vi "Counter - Count Edges AVG.vi"(6 "zero lag +":i32=1, 8 "AC length":i32, 10 "Sample Rate":dbl=100000.0, 11 "Total Time (s)":i32=100) -> (1 "G2 MultipTau":dbl[][](graph), 2 "output params":T1, 3 "N":i32, 5 "Cancel Button out":bool)   [LabVIEW 2022 SP3]
doc: "This example demonstrates how to continuously read back the number of digital edges that have been counted by a counter input. It uses an external clock so that the samples of the count register occur at regular intervals. If you do not need deterministic sampling of the count register, refer instead to the Count Edges example which does not use an external clock.\n\nFor instructions on how to connect your signals to the DAQ device, refer to your device documentation."
uses:
  <vilib>/DAQmx/read.llb/DAQmx Read (Counter 1D U32 1Chan NSamp).vi
  <vilib>/DAQmx/create/channels.llb/DAQmx Create Channel (CO-Pulse Generation-Frequency).vi
  <vilib>/DAQmx/configure/timing.llb/DAQmx Timing (Implicit).vi
  <vilib>/DAQmx/create/channels.llb/DAQmx Create Channel (CI-Count Edges).vi
  <vilib>/DAQmx/configure/timing.llb/DAQmx Timing (Sample Clock).vi
  <vilib>/DAQmx/miscellaneous.llb/DAQmx Fill In Error Info.vi
  <resource>/objmgr/daqmx.rc
panel:
  out "Current N":i32
  in  "Cancel Button":bool
  in  "Input Terminal":tag="/Dev1/PFI3"
  in  "Counter":tag="Dev1/ctr1"
  in  "Sample Clock Source":tag="/Dev1/PFI12"
  # "Channel Settings"
  # "Timing Settings"
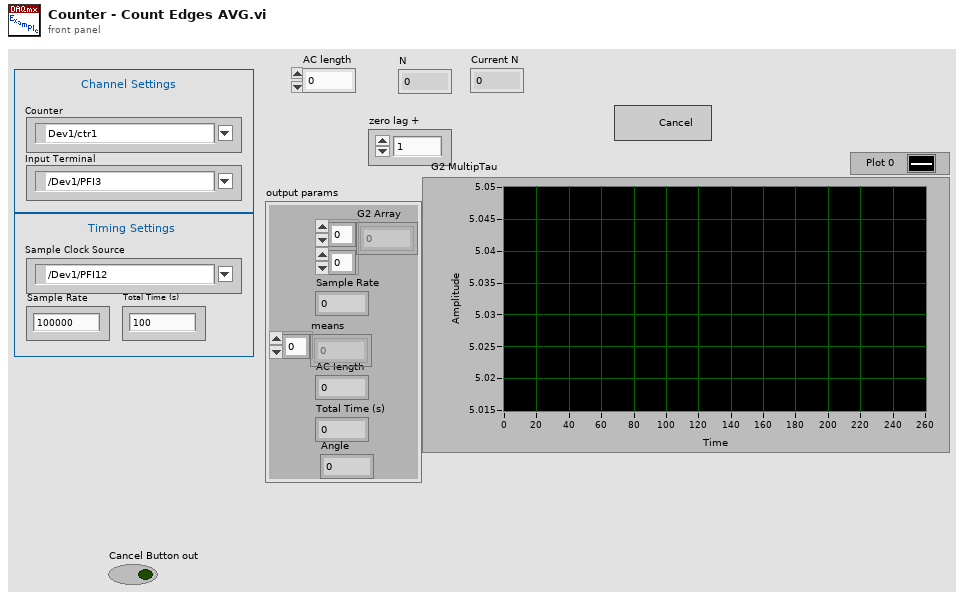
[diagram p1: front panel]
types:
  T1 = cluster{"G2 Array":dbl[][], "Sample Rate":dbl, "means":dbl[], "AC length":i32, "Total Time (s)":i32, "Angle":dbl}
  T2 = cluster{"Data out":dbl[][], "Sample Rate":dbl, dbl[], "AC length":i32, "Total Time (s)":i32, "AC length":dbl}
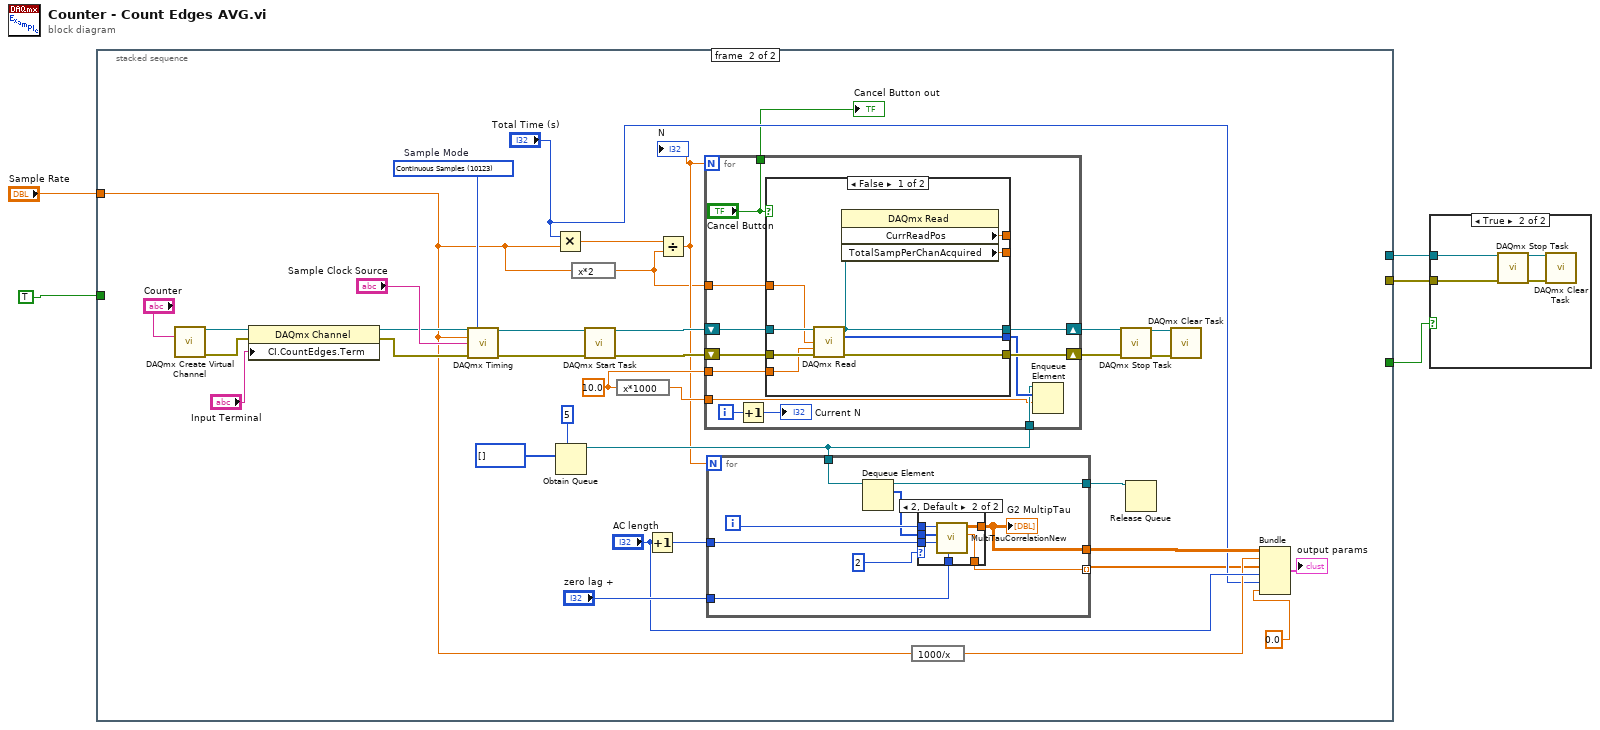
[diagram p0: block diagram]
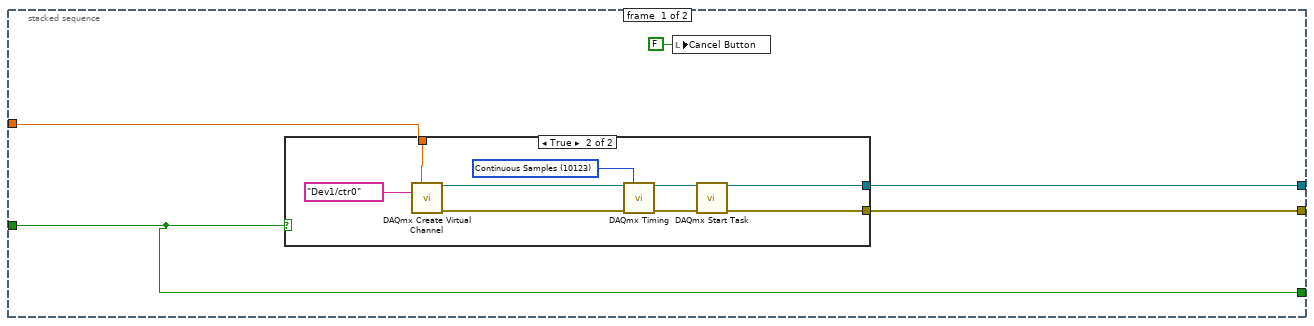
[diagram p2: hidden frame]
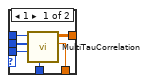
[diagram p4: hidden frame]
diagram:
  n1 = stacked-sequence {
    tunnel: TRUE -> [w6 _]
    tunnel: "Sample Rate" -> [w8 w22]
    tunnel: [w10 _] -> w4
    tunnel: [w9 _] -> w3
    tunnel: [w6 _] -> w1
    frame #0 {
      n2 = case shown="True" w6 {
        tunnel: w8 -> [_ w19]
        tunnel: [_ w17] -> w10
        tunnel: [_ w16] -> w9
        frame False {
        }
        frame True {
          w13 = 10123 items=["Finite Samples"=10178, "Continuous Samples"=10123, "Hardware Timed Single Point"=12522] ("sample mode")
          n3 = call-poly <vilib>:"DAQmx Create Virtual Channel.vi"("frequency"=w19, "counter"=tag "Dev1/ctr0") -> ("task out"=w15:refnum<k21>, "error out"=w12:errorcluster)  [unwired: 12 in]
          n4 = call-poly <vilib>:"DAQmx Timing.vi"("task/channels in"=w15, "sample mode"=w13, "error in"=w12) -> ("task out"=w14:refnum<k21>, "error out"=w11:errorcluster)  [unwired: 11 in]
          n5 = call <vilib>:"DAQmx Start Task.vi"("task/channels in"=w14, "error in"=w11) -> ("task out"=w17:refnum<k21>, "error out"=w16:errorcluster)  [unwired: 12 in]
        }
      }
      n6 = local write "Cancel Button"(FALSE ("Cancel Button")) -> ()
    }
    frame #1 {
      w34 = 10.0 ("timeout")
      w50 = 10123 items=["Finite Samples"=10178, "Continuous Samples"=10123, "Hardware Timed Single Point"=12522]  # Sample Mode
      n7 = call-poly <vilib>:"DAQmx Create Virtual Channel.vi"("counter"="Counter") -> ("task out"=w49:refnum<k21>, "error out"=w46:errorcluster)  [unwired: 13 in]
      n8 = property class="DAQmx Channel"(reference=w49, error in=w46, "CI.CountEdges.Term"="Input Terminal") -> (reference out=w48:refnum<k21>, error out=w47:errorcluster)
      n9 = call-poly <vilib>:"DAQmx Timing.vi"("task/channels in"=w48, "sample mode"=w50, "rate"=w22, "source"="Sample Clock Source", "error in"=w47) -> ("task out"=w44:refnum<k21>, "error out"=w45:errorcluster)  [unwired: 9 in]
      n10 = Multiply(x="Total Time (s)", y=w22) -> (x*y=w32:dbl)
      n11 = Obtain Queue(max queue size (-1, unlimited)=5, element data type=u32[] [] ("data")) -> (queue out=w36:refnum<queue>)  [unwired: 3 in, 2 out]
      n12 = expression code="x*2"(w22) -> (w20:dbl)
      n13 = call <vilib>:"DAQmx Start Task.vi"("task/channels in"=w44, "error in"=w45) -> ("task out"=w43:refnum<k21>, "error out"=w42:errorcluster)  [unwired: 12 in]
      n14 = expression code="x*1000"(w34) -> (w35:dbl)
      n15 = Increment(x="AC length") -> (x+1=w30:i32)
      n16 = Divide(x=w32, y=w20) -> (x/y=w31:dbl)
      "N" <- w31
      n17 = for {
        N: w31 -> [_]
        shift-right: [w82] -> w41
        shift-left: w43 -> [w86]
        shift-right: [w87] -> w40
        shift-left: w42 -> [w88]
        tunnel: w36 -> [w84]
        tunnel: w35 -> [w83]
        tunnel: w34 -> [w81]
        tunnel: w20 -> [w80]
        tunnel: ["Cancel Button"] -> w21
        i -> [w79]
        n18 = Increment(x=w79) -> (x+1=→"Current N":i32)
        n19 = case shown="False" "Cancel Button" {
          tunnel: w88 -> [w97 w98]
          tunnel: [w96 w98] -> w87
          tunnel: w86 -> [w95 w99]
          tunnel: [w94 _] -> w85
          tunnel: [w93 w99] -> w82
          tunnel: w81 -> [w91 _]
          tunnel: w80 -> [w92 _]
          tunnel: [w90 _] -> _
          tunnel: [w89 _] -> _
          frame False {
            n20 = call-poly <vilib>:"DAQmx Read.vi"("task/channels in"=w95, "number of samples per channel"=w92, "timeout"=w91, "error in"=w97) -> ("task out"=w93:refnum<k21>, "data"=w94:u32[], "error out"=w96:errorcluster)  [unwired: 9 in]
            n21 = property class="DAQmx Read"(reference=w93) -> ("CurrReadPos"=w90:dbl, "TotalSampPerChanAcquired"=w89:dbl)  [unwired: 1 in, 2 out]
          }
          frame True {
          }
        }
        n22 = Enqueue Element(queue=w84, element=w85, timeout in ms (-1)=w83) -> ()  [unwired: 1 in, 3 out]
      }
      "Cancel Button out" <- w21
      n23 = for {
        N: w31 -> [_]
        tunnel: [w63] -> w24 mode=indexing
        tunnel: "zero lag +" -> [w62]
        tunnel: w30 -> [w61]
        tunnel: w36 -> [w60]
        tunnel: [w58] -> w33
        tunnel: [w56] -> w29
        i -> [w64]
        n24 = Dequeue Element(queue=w60) -> (queue out=w58:refnum<queue>, element=w59:u32[])  [unwired: 2 in, 2 out]
        n25 = case shown="2, Default" 2 {
          tunnel: w64 -> [w70 w76]
          tunnel: [w69 w75] -> w63
          tunnel: w62 -> [w68 w74]
          tunnel: w61 -> [w67 w73]
          tunnel: w59 -> [w66 w72]
          tunnel: [w65 w71] -> w56
          frame 1 {
            n26 = call "MultiTauCorrelation.vi"("zero lag +"=w68, "AC final pts"=w67, "counts"=w66, "First Call"=w70) -> ("Mean of  Bins"=w69:dbl, "Data out"=w65:dbl[][])  [unwired: 6 in]
          }
          frame 2, Default {
            n27 = call "MultiTauCorrelationNew.vi"("zero lag +"=w74, "AC final pts"=w73, "counts"=w72, "First Call"=w76) -> ("Mean of  Bins"=w75:dbl, "Data out"=w71:dbl[][])  [unwired: 6 in]
          }
        }
        "G2 MultipTau" <- w56
      }
      n28 = expression code="1000/x"(w22) -> (w27:dbl)
      n29 = call <vilib>:"DAQmx Stop Task.vi"("task/channels in"=w41, "error in"=w40) -> ("task out"=w52:refnum<k21>, "error out"=w51:errorcluster)  [unwired: 12 in]
      n30 = Release Queue(queue=w33) -> ()  [unwired: 2 in, 3 out]
      n31 = call <vilib>:"DAQmx Clear Task.vi"("task in"=w52, "error in"=w51) -> ()  [unwired: 13 in, 1 out]
      n32 = Bundle("Data out"=w29, "Sample Rate"=w27, w24, "AC length"="AC length", "Total Time (s)"="Total Time (s)", "AC length"=0.0) -> (→"output params":T2)  [unwired: 1 in]
    }
  }
  n33 = case shown="True" w1 {
    tunnel: w4 -> [_ w103]
    tunnel: w3 -> [_ w102]
    frame False {
    }
    frame True {
      n34 = call <vilib>:"DAQmx Stop Task.vi"("task/channels in"=w103, "error in"=w102) -> ("task out"=w101:refnum<k21>, "error out"=w100:errorcluster)  [unwired: 12 in]
      n35 = call <vilib>:"DAQmx Clear Task.vi"("task in"=w101, "error in"=w100) -> ()  [unwired: 13 in, 1 out]
    }
  }
